vi "Set DDG Address.vi"(6 "address":u8, 7 "t3":u8, 8 "error in (no error)":errorcluster, 9 "t2":u8, 10 "t1":u8, 11 "t0":u8) -> (0 "error out":errorcluster, 3 "function return":u32)   [LabVIEW 2014, in "atmcd32d.lvlib"]
doc: "unsigned int WINAPI SetDDGAddress(BYTE t0, BYTE t1, BYTE t2, BYTE t3, BYTE address);"
uses:
  atmcd32d.lvlib
  atmcd32d.dll
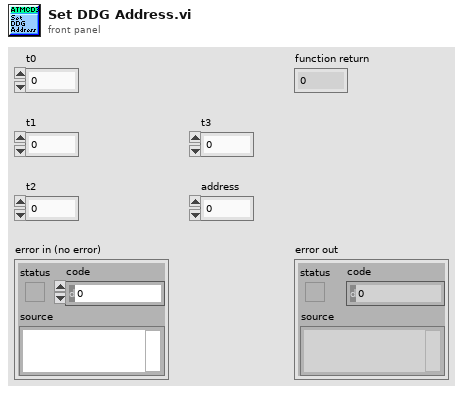
[diagram p1: front panel]
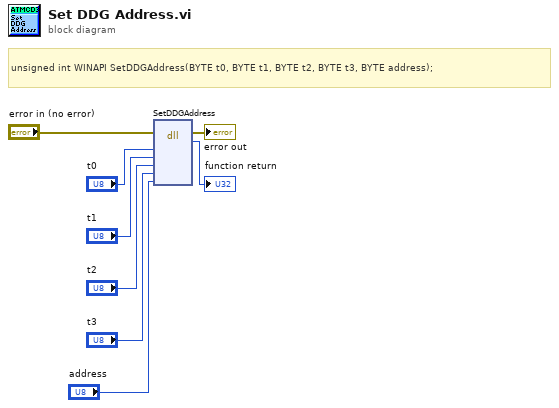
[diagram p0: block diagram]
diagram:
  # "unsigned int WINAPI SetDDGAddress(BYTE t0, BYTE t1, BYTE t2, BYTE t3, BYTE address);"
  n1 = dll-call lib="C:/Users/Bakir/Documents/Lambda2-Testing/lib/Andorlib/atmcd32d.*" fn="SetDDGAddress"(error in="error in (no error)", "t0"="t0", "t1"="t1", "t2"="t2", "t3"="t3", "address"="address") -> (error out=→"error out":errorcluster, →"function return":u32)  [unwired: 7 in, 1 out]
